vi "LSX Set TVR Mode.vi"(6 "lAT":i32, 7 "lZT":i32, 8 "error in (no error)":errorcluster, 9 "lYT":i32, 10 "lXT":i32, 11 "lLSID":i32) -> (0 "error out":errorcluster, 3 "function return":i32)   [LabVIEW 2016, in "Tango_DLL.lvlib"]
doc: "TANGOAPI int TANGOCALL LSX_SetTVRMode (int lLSID, int lXT, int lYT, int lZT, int lAT);"
uses:
  Tango_DLL.lvlib
  2017/Microscope Control/Device Library/Stages/Marzhauser/SCAN IM 120 x 80/Tango DLL VIs/Tango_DLL.dll
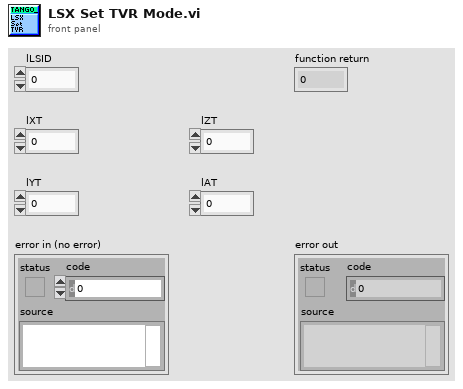
[diagram p1: front panel]
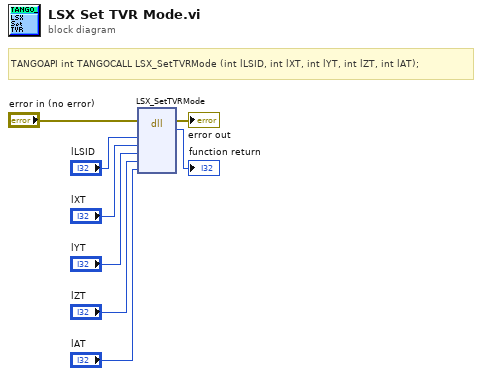
[diagram p0: block diagram]
diagram:
  # "TANGOAPI int TANGOCALL LSX_SetTVRMode (int lLSID, int lXT, int lYT, int lZT, int lAT);"
  n1 = dll-call lib="C:/Users/4PiSMS/Documents/Microscope Control/2017/Microscope Control/Device Library/Stages/Marzhauser/SCAN IM 120 x 80/Tango DLL VIs/Tango_DLL.*" fn="LSX_SetTVRMode"(error in="error in (no error)", "lLSID"="lLSID", "lXT"="lXT", "lYT"="lYT", "lZT"="lZT", "lAT"="lAT") -> (error out=→"error out":errorcluster, →"function return":i32)  [unwired: 7 in, 1 out]
